vi "UTL_Read_Write Controllers.vi"(8 "error in":errorcluster) -> (0 "error out":errorcluster, 2 "StatusCtrl":T1(array[cluster]), 5 "Results":dbl[][][](array[numeric]))   [LabVIEW 2019]
uses:
  <vilib>/Plasmionique/MB Master/MB_Master_Serial/MB_Master_Serial.lvclass
  C:/Program Files (x86)/National Instruments/LabVIEW 2024/vi.lib/Plasmionique/MB Master/MB_Master/MB_Master.lvclass
  Variable global de carga.vi
  <vilib>/Plasmionique/MB Master/MB Master.lvlib
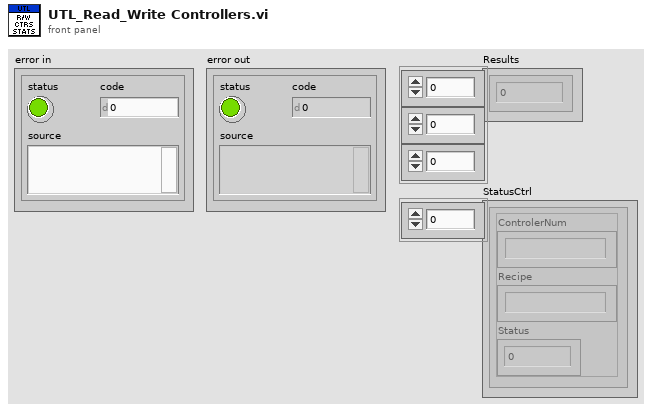
[diagram p1: front panel]
types:
  T1 = cluster{"ControlerNum":string, "Recipe":string, "Status":u32}[]
  T2 = typedef "Control 2.ctl" = refnum<class "MB_Master_Serial.lvclass">[]
  T3 = cluster{"ControlerNum":string, "Recipe":string, "Status":u32}
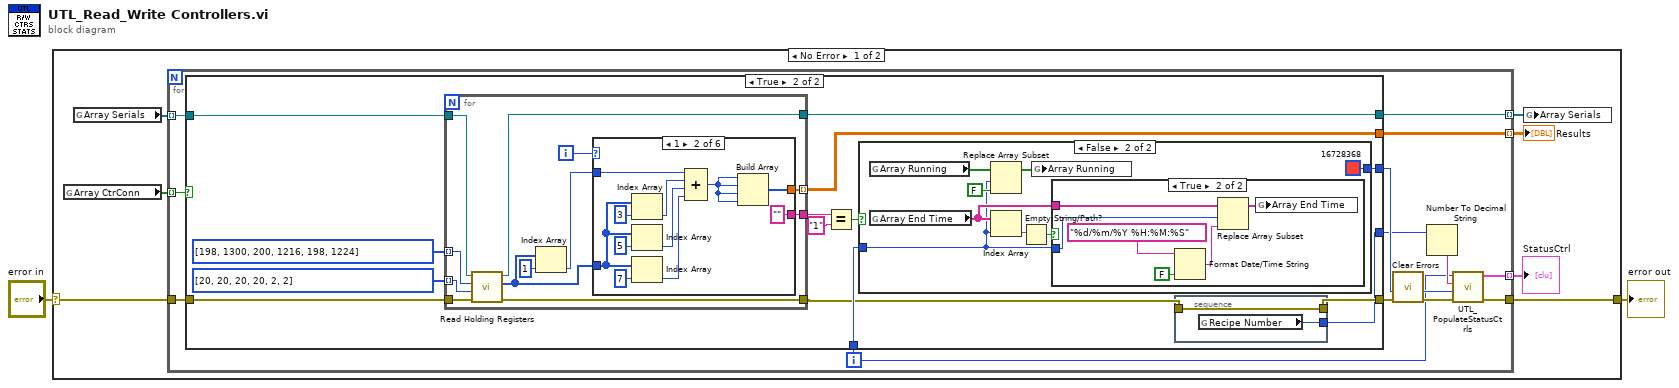
[diagram p0: block diagram]
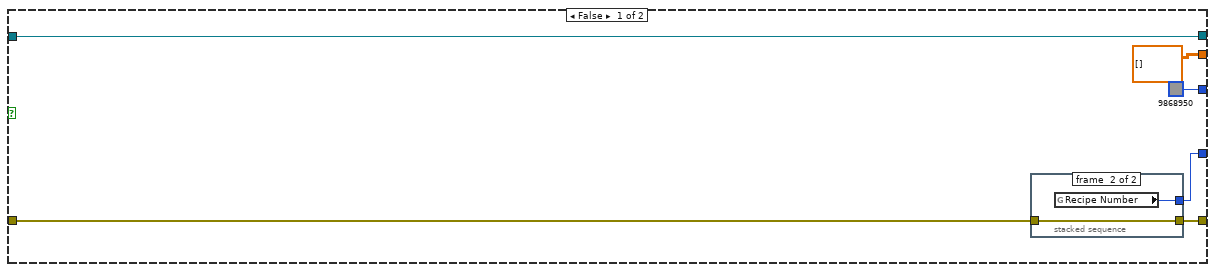
[diagram p2: hidden frame]
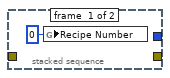
[diagram p3: hidden frame]
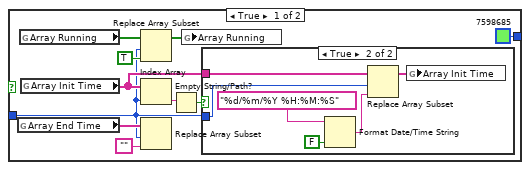
[diagram p4: hidden frame]
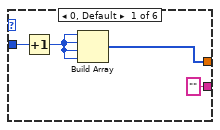
[diagram p7: hidden frame]
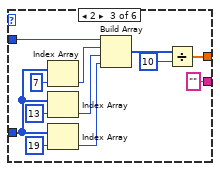
[diagram p8: hidden frame]
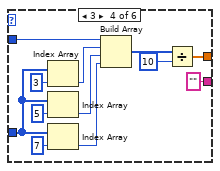
[diagram p9: hidden frame]
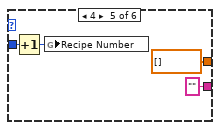
[diagram p10: hidden frame]
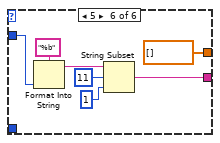
[diagram p11: hidden frame]
diagram:
  n1 = case shown="No Error" "error in" {
    selector: "error in" -> [w8 w140]
    tunnel: [w9 w140] -> w1
    frame No Error {
      n2 = global read "Variable global de carga.vi" "Array CtrConn"() -> (w3:bool[])
      n3 = global read "Variable global de carga.vi" "Array Serials"() -> (w7:T2)
      n4 = for {
        tunnel: w7 -> [w21] mode=indexing
        tunnel: [w20] -> w6 mode=indexing
        tunnel: [w19] -> w5 mode=indexing
        tunnel: w8 -> [w22]
        tunnel: [w18] -> w9
        tunnel: [w17] -> w4 mode=indexing
        tunnel: w3 -> [w11] mode=indexing
        i -> [w12]
        n5 = case shown="True" w11 {
          tunnel: w22 -> [w23 w45]
          tunnel: w21 -> [w28 w40]
          tunnel: [w28 w39] -> w20
          tunnel: [dbl[][] [] w32] -> w19
          tunnel: w12 -> [_ w37]
          tunnel: [w24 w34] -> w14
          tunnel: [u32 9868950 ("Status") w36] -> w13
          tunnel: [w25 w33] -> w10
          frame False {
            n6 = stacked-sequence {
              tunnel: [_ w31] -> w25
              tunnel: [_ w30] -> w24
              tunnel: w23 -> [_ w30]
              frame #0 {
                n7 = global write "Variable global de carga.vi" "Recipe Number"(u16 0 ("Recipe Number")) -> ()
              }
              frame #1 {
                n8 = global read "Variable global de carga.vi" "Recipe Number"() -> (w31:u16)
              }
            }
          }
          frame True {
            n9 = for {
              tunnel: i32[] [198, 1300, 200, 1216, 198, 1224] -> [w85] mode=indexing
              tunnel: [w88] -> w39
              tunnel: [w89] -> w35
              tunnel: [w86] -> w32 mode=indexing
              tunnel: i32[] [20, 20, 20, 20, 2, 2] -> [w84] mode=indexing
              tunnel: w45 -> [w80]
              tunnel: w40 -> [w79]
              tunnel: [w78] -> w41
              i -> [w87]
              n10 = call <vilib>:"Read Holding Registers.vi"("error in (no error)"=w80, "quantity"=w84, "starting address"=w85, "MB session in"=w79) -> ("error out"=w89:errorcluster, "Registers"=w81:u16[], "MB session out"=w88:refnum<class "MB_Master_Serial.lvclass">)  [unwired: 5 in]
              n11 = Index Array(array=w81, index=1) -> (element=w82:u16)
              n12 = case shown="1" w87 {
                tunnel: w81 -> [_ w101 w113 w125 _ _]
                tunnel: [w92 w96 w107 w119 dbl[] [] dbl[] []] -> w86
                tunnel: w82 -> [w91 w95 w106 w118 w132 w135]
                tunnel: ["" "" "" "" "" w133] -> w78
                frame 0, Default {
                  n13 = Increment(x=w91) -> (x+1=w93:u16)
                  n14 = Build Array(w93, w93, w93, w93) -> (w92:u16[])
                }
                frame 1 {
                  n15 = Index Array(array=w101, index=3) -> (element=w100:u16)
                  n16 = Index Array(array=w101, index=5) -> (element=w99:u16)
                  n17 = Index Array(array=w101, index=7) -> (element=w98:u16)
                  n18 = Compound Arithmetic op=ADD(w95, w100, w99, w98) -> (w97:u16)
                  n19 = Build Array(w97, w97, w97, w97) -> (w96:u16[])
                }
                frame 2 {
                  n20 = Index Array(array=w113, index=7) -> (element=w112:u16)
                  n21 = Index Array(array=w113, index=13) -> (element=w111:u16)
                  n22 = Index Array(array=w113, index=19) -> (element=w110:u16)
                  n23 = Build Array(w106, w112, w111, w110) -> (w108:u16[])
                  n24 = Divide(x=w108, y=10) -> (x/y=w107:dbl[])
                }
                frame 3 {
                  n25 = Index Array(array=w125, index=3) -> (element=w124:u16)
                  n26 = Index Array(array=w125, index=5) -> (element=w123:u16)
                  n27 = Index Array(array=w125, index=7) -> (element=w122:u16)
                  n28 = Build Array(w118, w124, w123, w122) -> (w120:u16[])
                  n29 = Divide(x=w120, y=10) -> (x/y=w119:dbl[])
                }
                frame 4 {
                  n30 = Increment(x=w132) -> (x+1=w129:u16)
                  n31 = global write "Variable global de carga.vi" "Recipe Number"(w129) -> ()
                }
                frame 5 {
                  n32 = Format Into String(format string="%b", w135) -> (resulting string=w139:string)  [unwired: 2 in, 1 out]
                  n33 = String Subset(string=w139, offset (0)=11, length (rest)=1 ("length (rest)")) -> (substring=w133:string)
                }
              }
            }
            n34 = Equal?(x=w41, y="1") -> (x = y?=w38:bool)
            n35 = case shown="False" w38 {
              tunnel: w37 -> [w49 w65]
              tunnel: [u32 7598685 ("Status 3") u32 16728368 ("Status 4")] -> w36
              frame True {
                n36 = global read "Variable global de carga.vi" "Array End Time"() -> (w51:string[])
                n37 = global read "Variable global de carga.vi" "Array Running"() -> (w53:bool[])
                n38 = global read "Variable global de carga.vi" "Array Init Time"() -> (w55:string[])
                n39 = Replace Array Subset(array=w53, new element=TRUE, index=w49) -> (w52:bool[])
                n40 = Index Array(array=w55, index=w49) -> (element=w57:string)
                n41 = Replace Array Subset(array=w51, new element="" ("new element/subarray"), index=w49) -> ()  [unwired: 1 out]
                n42 = Empty String/Path?(string/path=w57) -> (empty?=w56:bool)
                n43 = global write "Variable global de carga.vi" "Array Running"(w52) -> ()
                n44 = case shown="True" w56 {
                  tunnel: w49 -> [_ w60]
                  tunnel: w55 -> [_ w61]
                  frame False {
                  }
                  frame True {
                    n45 = Format Date/Time String(time format string (%c)="%d/%m/%Y %H:%M:%S", UTC format=FALSE) -> (date/time string=w58:string)  [unwired: 1 in]
                    n46 = Replace Array Subset(array=w61, new element=w58, index=w60) -> (w59:string[])
                    n47 = global write "Variable global de carga.vi" "Array Init Time"(w59) -> ()
                  }
                }
              }
              frame False {
                n48 = global read "Variable global de carga.vi" "Array Running"() -> (w67:bool[])
                n49 = global read "Variable global de carga.vi" "Array End Time"() -> (w69:string[])
                n50 = Replace Array Subset(array=w67, new element=FALSE, index=w65) -> (w66:bool[])
                n51 = Index Array(array=w69, index=w65) -> (element=w71:string)
                n52 = Empty String/Path?(string/path=w71) -> (empty?=w70:bool)
                n53 = global write "Variable global de carga.vi" "Array Running"(w66) -> ()
                n54 = case shown="True" w70 {
                  tunnel: w65 -> [_ w74]
                  tunnel: w69 -> [_ w75]
                  frame False {
                  }
                  frame True {
                    n55 = Format Date/Time String(time format string (%c)="%d/%m/%Y %H:%M:%S", UTC format=FALSE) -> (date/time string=w72:string)  [unwired: 1 in]
                    n56 = Replace Array Subset(array=w75, new element=w72, index=w74) -> (w73:string[])
                    n57 = global write "Variable global de carga.vi" "Array End Time"(w73) -> ()
                  }
                }
              }
            }
            n58 = stacked-sequence {
              tunnel: [w47] -> w33
              tunnel: w35 -> [w46]
              tunnel: [w46] -> w34
              frame #0 {
                n59 = global read "Variable global de carga.vi" "Recipe Number"() -> (w47:u16)
              }
            }
          }
        }
        n60 = call <vilib>:"Clear Errors.vi"("error in (no error)"=w14) -> ("error out"=w15:errorcluster)  [unwired: 5 in, 1 out]
        n61 = Number To Decimal String(number=w10) -> (decimal integer string=w16:string)  [unwired: 1 in]
        n62 = call "UTL_PopulateStatusCtrls.vi"("error in (no error)"=w15, "Status"=w13, "Recipe"=w16, "ComNum"=w12) -> ("error out"=w18:errorcluster, "output cluster"=w17:T3)  [unwired: 6 in]
      }
      "Results" <- w5
      "StatusCtrl" <- w4
      n63 = global write "Variable global de carga.vi" "Array Serials"(w6) -> ()
    }
    frame Error {
    }
  }
  "error out" <- w1
